vi "full_rt_layer.vi"() -> ()   [LabVIEW 2014]
uses:
  <vilib>/LabVIEW Targets/FPGA/cRIO/cRIO-9505/controls.llb/_nicrio_cRIO-9505_DriveStatus.ctl
  <vilib>/FPGAPlugInAG/cRIO-9074/niLvFpga_Open_cRIO-9074.vi
  <vilib>/Utility/error.llb/Error Cluster From Error Code.vi
  <vilib>/rvi/errors/niLvFpgaAdjustHostInterfaceError.vi
  <vilib>/FPGAPlugInAG/cRIO-9074/niLvFpga_Close_cRIO-9074.vi
  <vilib>/rvi/interface/nirviOpenFPGA/nirviOpenFPGA.xnode
  FPGA Bitfiles/MotorLabAProject_FPGATarget_fullfpgalayer_geeQA2EZIvY.lvbitx
  full_fpga_layer.vi
  <vilib>/rvi/interface/nirviReadWriteControl/nirviReadWriteControl.xnode
  <vilib>/rvi/interface/nirviCloseFPGA/nirviCloseFPGA.xnode
  NiFpgaLv.dll
panel:
  in  "Degree":i32
  out "Analog PID Gains Debug":T1
  out "Analog Debug Desired Position Setpoint (Counts)":i32
  out "output cluster":T2
  in  "Analog Desired \nPosition Setpoint \n(Counts)":i32
  in  "Count(uSec)":u32
  out "PWM Current  Command":i16
  out "Analog PID Scaled Output":fxp<+/-,34,17>
  in  "Reset Analog Counter":bool
  out "Set Point in Counts":dbl
  out "Waveform Chart 2":cluster{dbl, i32}(graph)
  out "Stepper Current (Steps)":i32
  out "Stepper Steps to move":i32
  in  "Reset Stepper Counter":bool
  out "PWM Angular Position":dbl
  out "Pot Angular \nPosition (deg)":fxp<+/-,33,11>
  out "error out":errorcluster
  in  "Position Loop  Rate (usec)":u16=250
  in  "Position Error Limit":i16=32767
  out "Position Error Read":i16
  out "Position Error Status":bool
  out "Encoder Position":i32
  in  "Reset Encoder Position":bool
  in  "stop":bool
  out "Drive Status":T3=enum."Disabled"
  out "Waveform Chart":cluster{i64, "PWM Encoder Position":i32}(graph)
  # "PWM SERVO"
  # "USE ESTOP!"
  # "ANALOG SERVO"
  # "STEPPER"
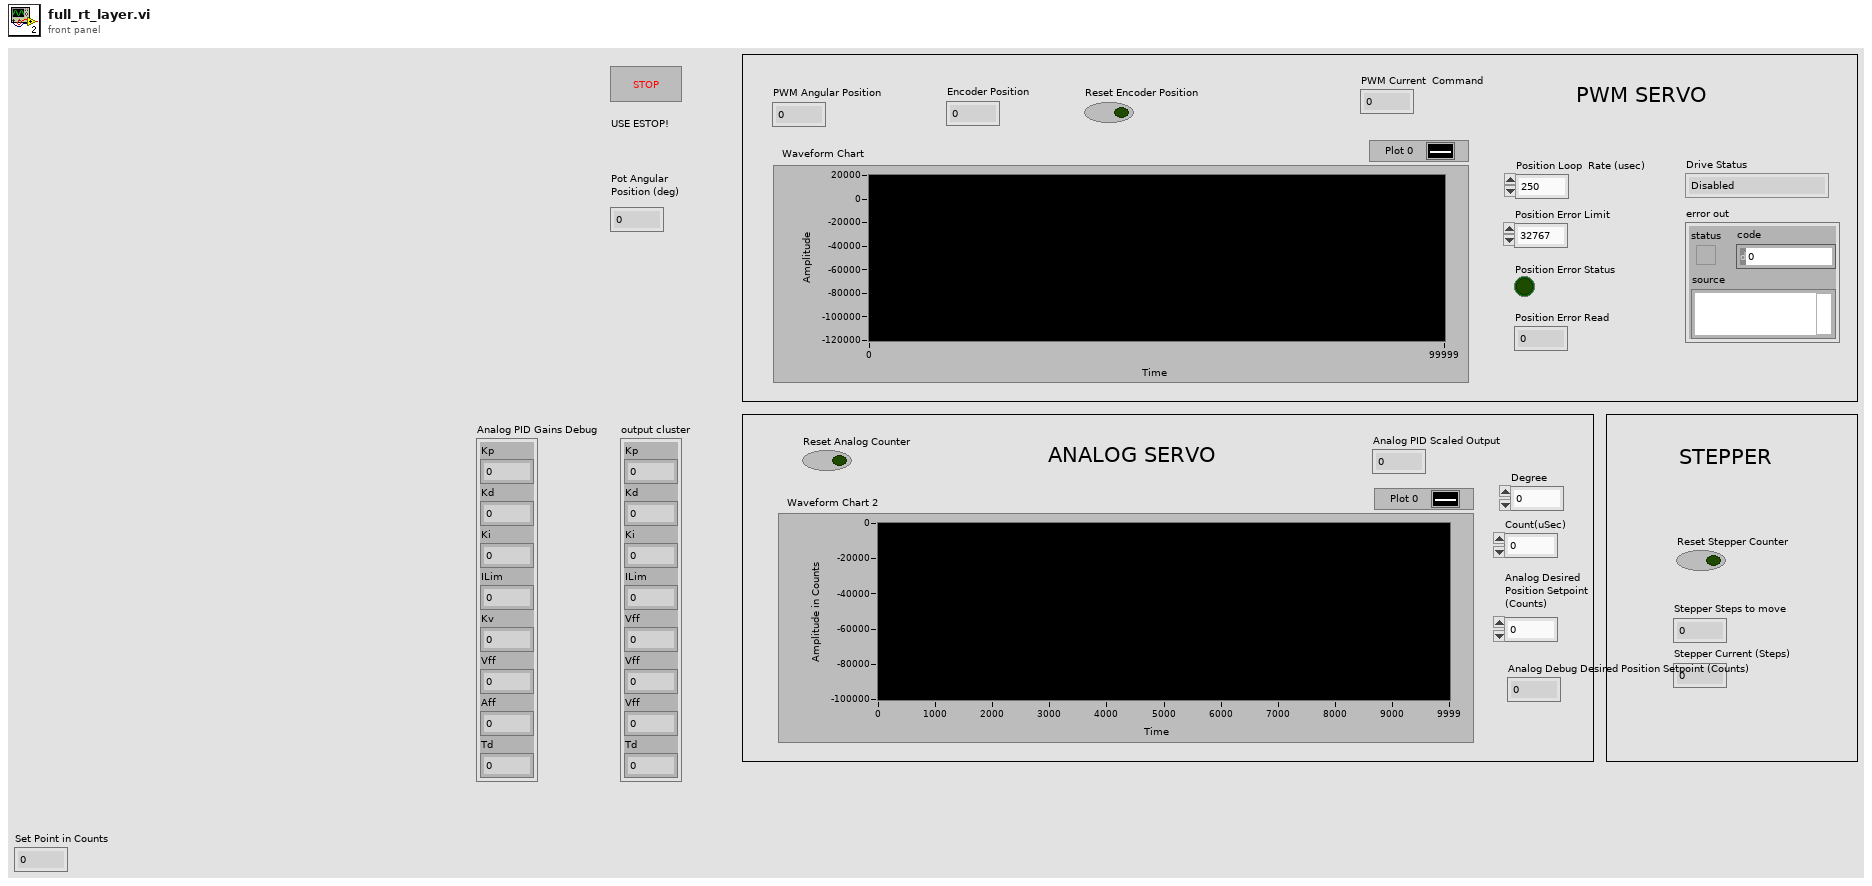
[diagram p1: front panel]
types:
  T1 = cluster{"Kp":i16, "Kd":i16, "Ki":i16, "ILim":i16, "Kv":i16, "Vff":i16, "Aff":i16, "Td":i16}
  T2 = cluster{"Kp":i16, "Kd":i16, "Ki":i16, "ILim":i16, "Vff":i16, "Vff":i16, "Vff":i16, "Td":i16}
  T3 = typedef "_nicrio_cRIO-9505_DriveStatus.ctl" = enum8{"Enabled", "Disabled", "Disabled by Drive Fault", "Disabled by Temp. Fault", "Disabled by E-Stop", "Unknown"}
  T4 = cluster{dbl, "Analog Position  Feedback (Counts)":i32}
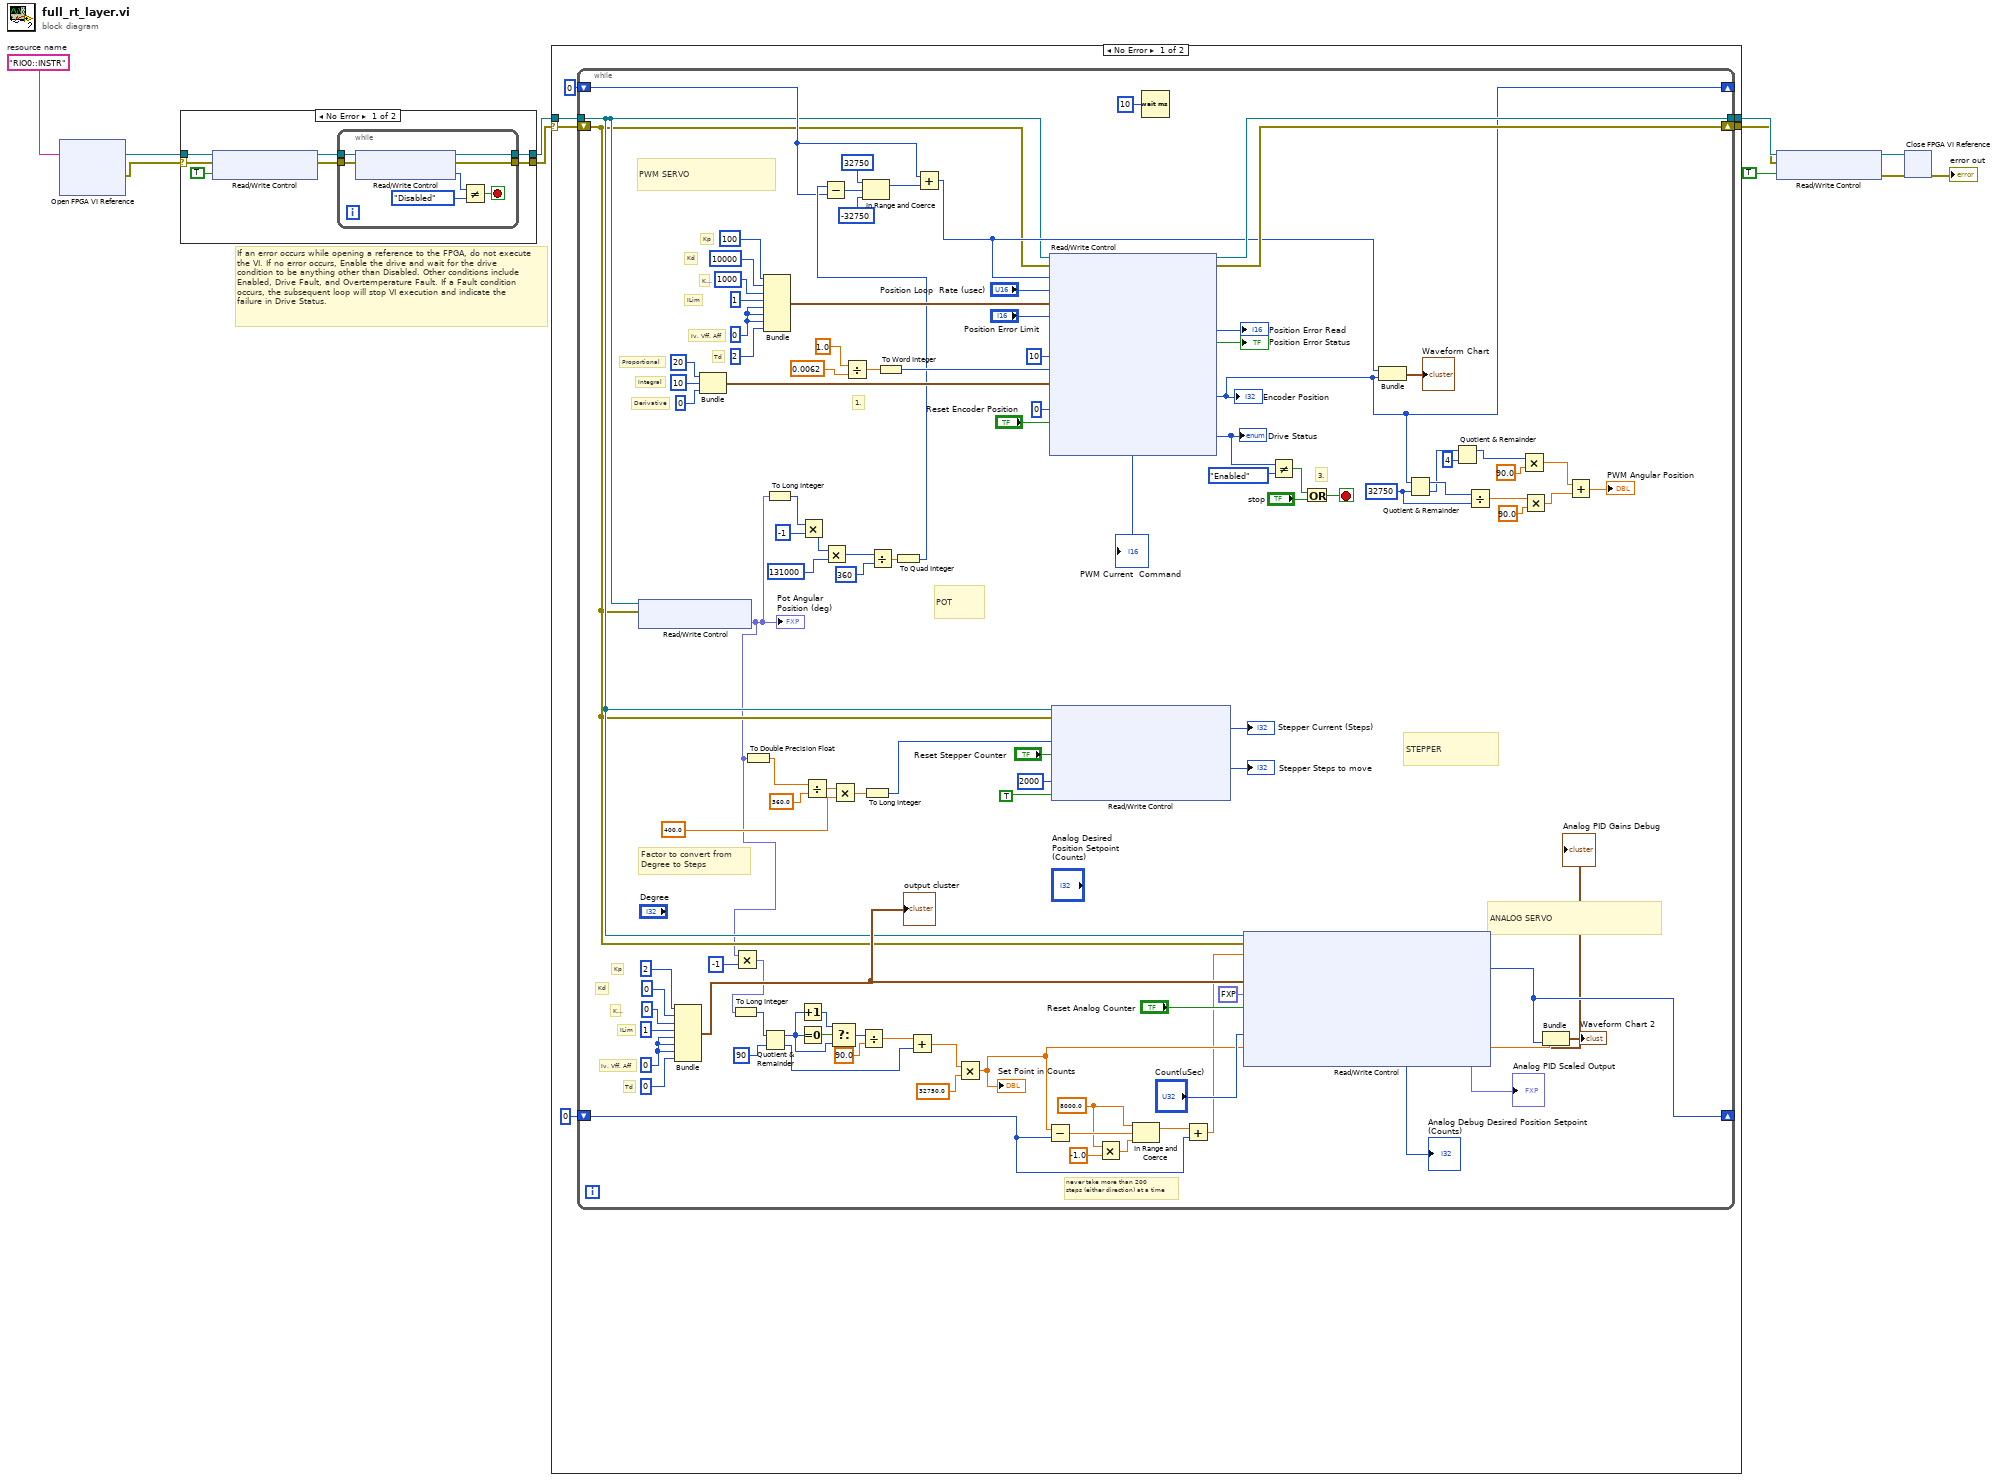
[diagram p0: block diagram]
diagram:
  w2 = "RIO0::INSTR"  # resource name
  # "If an error occurs while opening a reference to the FPGA, do not execute the VI. If no error occurs, Enable the drive and wait for the drive condition to be anything other than Disabled. Other conditions include Enabled, Drive Fault, and Overtemperature Fault. If a Fault condition occurs, the subsequent loop will stop VI execution and indicate the failure in Drive Status."
  n1 = xnode "Open FPGA VI Reference"("resource name"=w2) -> ("FPGA VI Reference Out"=w5:refnum<k20>, "error out"=w4:errorcluster)  [unwired: 1 in]
  n2 = case shown="No Error" w4 {
    selector: w4 -> [w13 w26]
    tunnel: w5 -> [w16 w27]
    tunnel: [w18 w27] -> w6
    tunnel: [w17 w26] -> w3
    frame No Error {
      n3 = xnode "Read/Write Control"("FPGA VI Reference In"=w16, "error in"=w13, "PWM  Enable Drive"=TRUE ("Enable Drive")) -> ("FPGA VI Reference Out"=w15:refnum<k20>, "error out"=w14:errorcluster)
      n4 = while {
        tunnel: [w25] -> w18
        tunnel: [w21] -> w17
        tunnel: w15 -> [w20]
        tunnel: w14 -> [w19]
        stop <- w22 stop-if-true
        n5 = xnode "Read/Write Control"("FPGA VI Reference In"=w20, "error in"=w19) -> ("FPGA VI Reference Out"=w25:refnum<k20>, "error out"=w21:errorcluster, "PWM Drive Status"=w24:T3)
        n6 = Not Equal?(x=w24, y=_nicrio_cRIO-9505_DriveStatus."Disabled") -> (x != y?=w22:bool)
      }
    }
    frame Error {
      # "Error occurred. Do not run."
    }
  }
  n7 = case shown="No Error" w3 {
    selector: w3 -> [w30 w142]
    tunnel: w6 -> [w33 w143]
    tunnel: [w32 w143] -> w11
    tunnel: [w31 w142] -> w10
    frame No Error {
      n8 = while {
        tunnel: w33 -> [w46]
        tunnel: [w137] -> w32
        shift-right: [w113] -> w31
        shift-left: w30 -> [w45]
        shift-right: [w92] -> _
        shift-left: 0 -> [w90]
        shift-right: [w48] -> _
        shift-left: 0 -> [w61]
        stop <- w114 stop-if-true
        w52 = 8000.0
        w71 = i16 0 ("Vff")
        w111 = 32750 ("y")
        w123 = i16 0 ("Vff")
        # "never take more than 200 \nsteps (either direction) at a time"
        # "ANALOG SERVO"
        # "STEPPER"
        # "POT"
        # "Td"
        # "Iv, Vff, Aff"
        # "ILim"
        # "Ki"
        # "Kd"
        # "Kp"
        # "Factor to convert from \nDegree to Steps"
        # "PWM SERVO"
        # "Derivative"
        # "Integral"
        # "Proportional"
        # "Td"
        # "Iv, Vff, Aff"
        # "ILim"
        # "Ki"
        # "Kd"
        # "Kp"
        # "3."
        # "1."
        n9 = xnode "Read/Write Control"("FPGA VI Reference In"=w46, "error in"=w45) -> ("Pot Angular Position"=w35:fxp<+/-,33,11>)  [unwired: 2 out]
        "Pot Angular \nPosition (deg)" <- w35
        n10 = Bundle("Kp"=i16 2, "Kd"=i16 0, "Ki"=i16 0, "ILim"=i16 1, "Vff"=w71, "Vff"=w71, "Vff"=w71, "Td"=i16 0) -> (w69:T2)  [unwired: 1 in]
        "output cluster" <- w69
        n11 = Bundle("Td"=i16 20, "Td"=i16 10, "Td"=i16 0) -> (w117:cluster{"Td":i16, "Td":i16, "Td":i16})  [unwired: 1 in]
        n12 = Multiply(x=w35, y=-1) -> (x*y=w34:fxp<+/-,64,42>)
        n13 = To Long Integer(number=w34) -> (32bit integer=w47:i32)
        n14 = To Double Precision Float(number=w35) -> (double precision float=w55:dbl)
        n15 = Quotient & Remainder(x=w47, y=90) -> (x-y*floor(x/y)=w58:i32, floor(x/y)=w51:i32)
        n16 = Bundle("Kp"=i16 100, "Kd"=i16 10000, "Ki"=i16 1000, "ILim"=i16 1, "Vff"=w123, "Vff"=w123, "Vff"=w123, "Td"=i16 2) -> (w121:T2)  [unwired: 1 in]
        n17 = To Long Integer(number=w35) -> (32bit integer=w89:i32)
        n18 = Increment(x=w58) -> (x+1=w57:i32)
        n19 = Equal To 0?(x=w58) -> (x = 0?=w59:bool)
        n20 = Multiply(x=w89, y=-1) -> (x*y=w88:i32)
        n21 = Divide(x=w55, y=360.0) -> (x/y=w86:dbl)
        n22 = Multiply(x=w88, y=131000) -> (x*y=w100:i32)
        n23 = Select(t=w57, s=w59, f=w58) -> (s? t:f=w56:i32)
        n24 = Multiply(x=w86, y=400.0) -> (x*y=w84:dbl)
        n25 = Divide(x=1.0, y=0.0062) -> (x/y=w133:dbl)
        n26 = Divide(x=w56, y=90.0) -> (x/y=w54:dbl)
        n27 = To Long Integer(number=w84) -> (32bit integer=w43:i32)
        n28 = Divide(x=w100, y=360) -> (x/y=w98:dbl)
        n29 = To Word Integer(number=w133) -> (16bit integer=w132:i16)
        n30 = To Quad Integer(1:w98) -> (0:w91:i64)
        n31 = Subtract(x=w91, y=w90) -> (x-y=w97:i64)
        n32 = In Range and Coerce(upper limit=i64 32750 ("lower limit"), x=w97, lower limit=i64 -32750) -> (coerced(x)=w94:i64)  [unwired: 1 out]
        n33 = Add(x=w54, y=w51) -> (x+y=w53:dbl)
        n34 = Add(x=w90, y=w94) -> (x+y=w93:i64)
        n35 = Multiply(x=w53, y=32750.0) -> (x*y=w41:dbl)
        "Set Point in Counts" <- w41
        n36 = Subtract(x=w41, y=w61) -> (x-y=w65:dbl)
        n37 = xnode "Read/Write Control"("FPGA VI Reference In"=w46, "error in"=w45, "PWM Position Setpoint"=w93, "PWM Position Loop  Rate (usec)"="Position Loop  Rate (usec)", "PWM Position PID Gains"=w121, "PWM Position Error Limit"="Position Error Limit", "PWM Current  Loop Rate (usec)"=u32 10, "PWM Current Limit"=w132, "PWM Current PI Gains"=w117, "PWM Reset Position Value"=0, "PWM Reset Position"="Reset Encoder Position") -> ("FPGA VI Reference Out"=w137:refnum<k20>, "error out"=w113:errorcluster, "PWM Position Error Read"=→"Position Error Read":i16, "PWM Position Error Status"=→"Position Error Status":bool, "PWM Encoder Position"=w92:i32, "PWM Drive Status"=w131:T3, "PWM Current  Command"=→"PWM Current  Command":i16)
        "Encoder Position" <- w92
        "Drive Status" <- w131
        n38 = xnode "Read/Write Control"("FPGA VI Reference In"=w46, "error in"=w45, "Stepper Desired Position (Steps)"=w43, "Stepper Reset Step Counter"="Reset Stepper Counter", "Stepper  Step Period (uS)"=i16 2000, "Stepper Enable/Disable Step Motor"=TRUE) -> ("Stepper Current (Steps)"=→"Stepper Current (Steps)":i32, "Stepper Steps to move"=→"Stepper Steps to move":i32)  [unwired: 2 out]
        n39 = Multiply(x=w52, y=-1.0) -> (x*y=w63:dbl)
        n40 = In Range and Coerce(upper limit=w52, x=w65, lower limit=w63) -> (coerced(x)=w62:dbl)  [unwired: 1 out]
        n41 = Wait (ms)(milliseconds to wait=u32 10) -> ()  [unwired: 1 out]
        n42 = Add(x=w62, y=w61) -> (x+y=w37:dbl)
        n43 = xnode "Read/Write Control"("FPGA VI Reference In"=w46, "error in"=w45, "Analog Desired Position Setpoint (Counts)"=w37, "Analog PID Gains"=w69, "Analog Shutdown Signal"=fxp<+/-,20,5> 2.5, "Analog Reset Enc"="Reset Analog Counter", "Analog Count(mSec)"="Count(uSec)") -> ("Analog Position  Feedback (Counts)"=w48:i32, "Analog PID Scaled Output"=→"Analog PID Scaled Output":fxp<+/-,34,17>, "Analog PID Gains Debug"=→"Analog PID Gains Debug":T1, "Analog Debug Desired Position Setpoint (Counts)"=→"Analog Debug Desired Position Setpoint (Counts)":i32)  [unwired: 2 out]
        n44 = Not Equal?(x=w131, y=_nicrio_cRIO-9505_DriveStatus."Enabled") -> (x != y?=w135:bool)
        n45 = Or(x=w135, y="stop") -> (x .or. y?=w114:bool)
        n46 = Bundle(w93, "PWM Encoder Position"=w92) -> (→"Waveform Chart":cluster{i64, "PWM Encoder Position":i32})  [unwired: 1 in]
        n47 = Quotient & Remainder(x=w92, y=w111) -> (x-y*floor(x/y)=w112:i32, floor(x/y)=w108:i32)
        n48 = Quotient & Remainder(x=w108, y=4) -> (x-y*floor(x/y)=w105:i32)  [unwired: 1 out]
        n49 = Divide(x=w112, y=w111) -> (x/y=w110:dbl)
        n50 = Multiply(x=w105, y=90.0) -> (x*y=w103:dbl)
        n51 = Multiply(x=w110, y=90.0) -> (x*y=w102:dbl)
        n52 = Bundle(w41, "Analog Position  Feedback (Counts)"=w48) -> (→"Waveform Chart 2":T4)  [unwired: 1 in]
        n53 = Add(x=w103, y=w102) -> (x+y=→"PWM Angular Position":dbl)
      }
    }
    frame Error {
      # "Error occurred. Do not run."
    }
  }
  n54 = xnode "Read/Write Control"("FPGA VI Reference In"=w11, "error in"=w10, "PWM Disable Drive"=TRUE ("Disable Drive")) -> ("FPGA VI Reference Out"=w9:refnum<k20>, "error out"=w8:errorcluster)
  n55 = xnode "Close FPGA VI Reference"("FPGA VI Reference In"=w9, "error in"=w8) -> ("error out"=→"error out":errorcluster)
